vi "剖面多参数上传.vi"(11 "错误输入（无错误）":errorcluster) -> (15 "error out":errorcluster)   [LabVIEW 2016, in "数据传输系统-05.lvlib"]
uses:
  <vilib>/Utility/config.llb/Write Key (String).vi
  <vilib>/Utility/config.llb/Read Key (String).vi
  <vilib>/Utility/config.llb/NI_LVConfig.lvlib
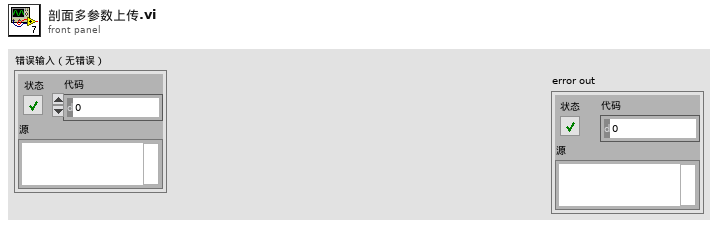
[diagram p1: front panel]
types:
  T1 = cluster{"setini":string, "sysini":string, "hechaini":string, "actualwrite":string, "actualread":string, "datasent":string, "反控命令信息队列":string, "反控与仪器交互":string}
  T2 = typedef "NI_LVConfig.lvlib/Config Data RefNum.ctl" = refnum<k1>
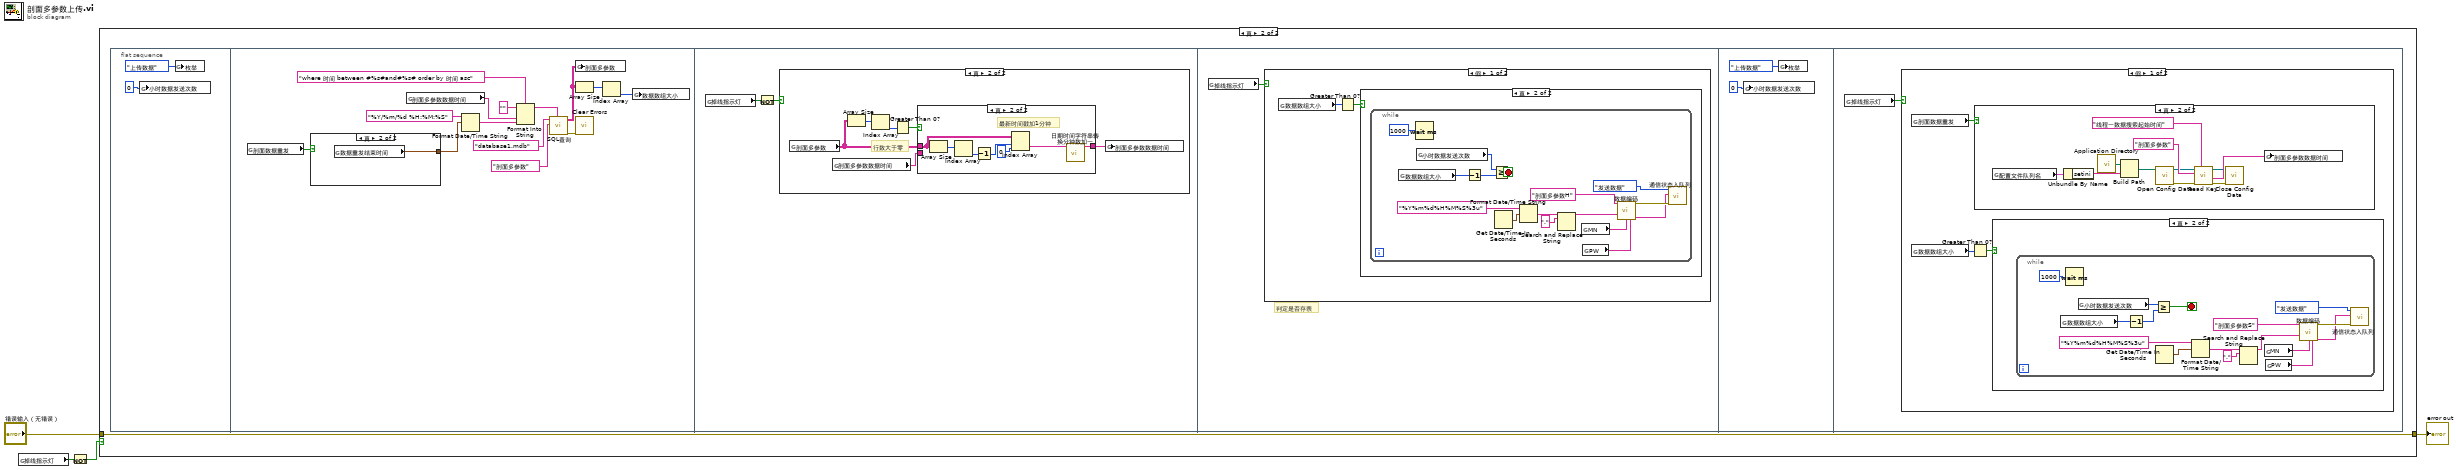
[diagram p0: block diagram]
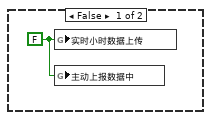
[diagram p2: hidden frame]
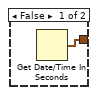
[diagram p3: hidden frame]
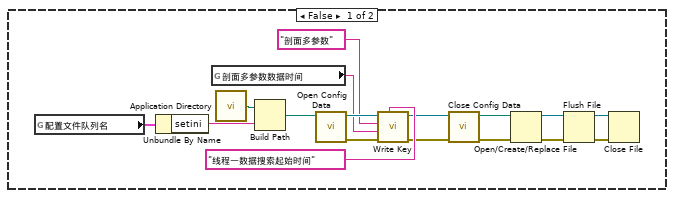
[diagram p8: hidden frame]
diagram:
  n1 = global read "全局 数据发送重叠.vi" "掉线指示灯"() -> (w4:bool)
  n2 = Not(x=w4) -> (.not. x?=w1:bool)
  n3 = case shown="真" w1 {
    tunnel: [_ w6] -> w3
    tunnel: "错误输入（无错误）" -> [_ w6]
    frame False {
      w5 = FALSE ("小时数据上传")
      n4 = global write "全局1.vi" "实时小时数据上传"(w5) -> ()
      n5 = global write "全局 数据发送重叠.vi" "主动上报数据中"(w5) -> ()
    }
    frame True {
      n6 = flat-sequence {
        frame #0 {
          n7 = global write "全局 小时数据发送次数.vi" "小时数据发送次数"(0 ("小时数据发送次数")) -> ()
          n8 = global write "全局1.vi" "枚举"(enum16{"返回请求应答", "上传数据", "返回执行结果"}."上传数据" ("枚举")) -> ()
        }
        frame #1 {
          n9 = global read "断电保存全局.vi" "剖面数据重发"() -> (w10:bool)
          n10 = case shown="真" w10 {
            tunnel: [w23 w24] -> w9
            frame False {
              n11 = Get Date/Time In Seconds() -> (seconds since 1Jan1904=w23:timestamp)
            }
            frame True {
              n12 = global read "断电保存全局.vi" "数据重发结束时间"() -> (w24:timestamp)
            }
          }
          n13 = global read "全局 水样时间.vi" "剖面多参数数据时间"() -> (w17:string)
          n14 = Format Date/Time String(time format string (%c)="%Y/%m/%d %H:%M:%S" ("时间格式字符串(%c)"), seconds (now)=w9) -> (date/time string=w16:string)  [unwired: 1 in]
          n15 = Format Into String(format string="where 时间 between #%s#and#%s# order by 时间 asc" ("condition"), initial string="" ("初始字符串"), w17, w16) -> (resulting string=w15:string)  [unwired: 1 in, 1 out]
          n16 = call "SQL查询.vi"("condition"=w15, "table输入"="剖面多参数", "database"="database1.mdb") -> ("error out"=w11:errorcluster, "data"=w14:string[][])  [unwired: 5 in, 2 out]
          n17 = global write "全局 所有参数.vi" "剖面多参数"(w14) -> ()
          n18 = Array Size(array=w14) -> (size(s)=w13:i32[])
          n19 = call <vilib>:"Clear Errors.vi"("error in (no error)"=w11) -> ()  [unwired: 5 in, 2 out]
          n20 = Index Array(array=w13) -> (element=w12:i32)  [unwired: 1 in]
          n21 = global write "全局 数据数组大小.vi" "数据数组大小"(w12) -> ()
        }
        frame #2 {
          n22 = global read "全局 数据发送重叠.vi" "掉线指示灯"() -> (w26:bool)
          n23 = Not(x=w26) -> (.not. x?=w25:bool)
          n24 = case shown="真" w25 {
            frame False {
            }
            frame True {
              # "行数大于零"
              n25 = global read "全局 所有参数.vi" "剖面多参数"() -> (w31:string[][])
              n26 = global read "全局 水样时间.vi" "剖面多参数数据时间"() -> (w32:string)
              n27 = Array Size(array=w31) -> (size(s)=w28:i32[])
              n28 = Index Array(array=w28) -> (element=w29:i32)  [unwired: 1 in]
              n29 = Greater Than 0?(x=w29) -> (x > 0?=w30:bool)
              n30 = case shown="真" w30 {
                tunnel: w31 -> [_ w37]
                tunnel: [w33 w34] -> w27
                tunnel: w32 -> [w33 _]
                frame False {
                }
                frame True {
                  # "最新时间戳加1分钟"
                  n31 = Array Size(array=w37) -> (size(s)=w39:i32[])
                  n32 = Index Array(array=w39) -> (element=w38:i32)  [unwired: 1 in]
                  n33 = Decrement(x=w38) -> (x-1=w36:i32)
                  n34 = Index Array(array=w37, index (row)=w36, index (col)=0 ("禁用的索引 (列)")) -> (element=w40:string)
                  n35 = call "日期时间字符串转换分钟数加一.vi"("data[0]"=w40) -> ("日期/时间字符串"=w34:string)  [unwired: 10 in]
                }
              }
              n36 = global write "全局 水样时间.vi" "剖面多参数数据时间"(w27) -> ()
            }
          }
        }
        frame #3 {
          # "判定是否存表"
          n37 = global read "全局 数据发送重叠.vi" "掉线指示灯"() -> (w41:bool)
          n38 = case shown="假" w41 {
            frame False {
              n39 = global read "全局 数据数组大小.vi" "数据数组大小"() -> (w42:i32)
              n40 = Greater Than 0?(x=w42) -> (x > 0?=w43:bool)
              n41 = case shown="真" w43 {
                frame False {
                }
                frame True {
                  n42 = while {
                    stop <- w46 stop-if-true
                    n43 = global read "全局 数据数组大小.vi" "数据数组大小"() -> (w48:i32)
                    n44 = Wait (ms)(milliseconds to wait=u32 1000 ("等待时间（毫秒）")) -> ()  [unwired: 1 out]
                    n45 = global read "全局 小时数据发送次数.vi" "小时数据发送次数"() -> (w49:i32)
                    n46 = Decrement(x=w48) -> (x-1=w47:i32)
                    n47 = Greater Or Equal?(x=w49, y=w47) -> (x >= y?=w46:bool)
                    n48 = Get Date/Time In Seconds() -> (seconds since 1Jan1904=w57:timestamp)
                    n49 = Format Date/Time String(time format string (%c)="%Y%m%d%H%M%S%3u" ("时间格式字符串(%c)"), seconds (now)=w57) -> (date/time string=w56:string)  [unwired: 1 in]
                    n50 = Search and Replace String(input string=w56, search string="." ("搜索字符串")) -> (result string=w54:string)  [unwired: 6 in, 3 out]
                    n51 = global read "断电保存全局.vi" "MN"() -> (w53:string)
                    n52 = global read "断电保存全局.vi" "PW"() -> (w52:string)
                    n53 = call "数据编码.vi"("table输入"="剖面多参数H" ("新元素/子数组"), "QN"=w54, "MN"=w53, "PW"=w52) -> ("错误常量"=w51:errorcluster, "通讯包字符串"=w44:string)  [unwired: 10 in]
                    n54 = call "通信状态入队列.vi"("错误输入（无错误）"=w51, "发送报文"=w44, "枚举"=enum16{"打开连接", "发送数据", "读取数据", "数据处理", "关闭连接"}."发送数据") -> ()  [unwired: 8 in, 1 out]
                  }
                }
              }
            }
            frame True {
            }
          }
        }
        frame #4 {
          n55 = global write "全局 小时数据发送次数.vi" "小时数据发送次数"(0 ("小时数据发送次数")) -> ()
          n56 = global write "全局1.vi" "枚举"(enum16{"返回请求应答", "上传数据", "返回执行结果"}."上传数据" ("枚举")) -> ()
        }
        frame #5 {
          n57 = global read "全局 数据发送重叠.vi" "掉线指示灯"() -> (w62:bool)
          n58 = case shown="假" w62 {
            frame False {
              n59 = global read "断电保存全局.vi" "剖面数据重发"() -> (w63:bool)
              n60 = global read "全局 数据数组大小.vi" "数据数组大小"() -> (w65:i32)
              n61 = Greater Than 0?(x=w65) -> (x > 0?=w64:bool)
              n62 = case shown="真" w63 {
                frame False {
                  n63 = global read "断电保存全局.vi" "配置文件队列名"() -> (w67:T1)
                  n64 = Unbundle By Name(w67) -> ("setini"=w66:string)
                  n65 = global read "全局 水样时间.vi" "剖面多参数数据时间"() -> (w68:string)
                  n66 = call <vilib>:"Application Directory.vi"() -> ("Application Directory"=w76:path)
                  n67 = Build Path(base path=w76, name or relative path=w66) -> (appended path=w77:path)
                  n68 = call <vilib>:"Open Config Data.vi"("configuration file path"=w77) -> ("error out"=w79:errorcluster, "refnum"=w78:T2)  [unwired: 8 in, 1 out]
                  n69 = call-poly <vilib>:"Write Key.vi"("section"="线程一数据搜索起始时间", "error in (no error)"=w79, "value"=w68, "key"="剖面多参数", "refnum"=w78) -> ("error out"=w81:errorcluster, "refnum out"=w80:T2)  [unwired: 4 in, 1 out]
                  n70 = call <vilib>:"Close Config Data.vi"("error in (no error)"=w81, "refnum"=w80) -> ("error out"=w69:errorcluster, "file path"=w70:path)  [unwired: 8 in]
                  n71 = Open/Create/Replace File(file path (use dialog)=w70, error in=w69) -> (refnum out=w72:refnum<file>, error out=w71:errorcluster)  [unwired: 4 in, 1 out]
                  n72 = Flush File(refnum=w72, error in=w71) -> (refnum out=w73:refnum<file>, error out=w74:errorcluster)
                  n73 = Close File(refnum=w73, error in=w74) -> ()  [unwired: 2 out]
                }
                frame True {
                  n74 = global read "断电保存全局.vi" "配置文件队列名"() -> (w89:T1)
                  n75 = Unbundle By Name(w89) -> ("setini"=w90:string)
                  n76 = call <vilib>:"Application Directory.vi"() -> ("Application Directory"=w88:path)
                  n77 = Build Path(base path=w88, name or relative path=w90) -> (appended path=w91:path)
                  n78 = call <vilib>:"Open Config Data.vi"("configuration file path"=w91) -> ("error out"=w85:errorcluster, "refnum"=w84:T2)  [unwired: 8 in, 1 out]
                  n79 = call-poly <vilib>:"Read Key.vi"("section"="线程一数据搜索起始时间", "error in (no error)"=w85, "key"="剖面多参数", "refnum"=w84) -> ("error out"=w87:errorcluster, "value"=w93:string, "refnum out"=w86:T2)  [unwired: 4 in, 1 out]
                  n80 = call <vilib>:"Close Config Data.vi"("error in (no error)"=w87, "refnum"=w86) -> ()  [unwired: 8 in, 2 out]
                  n81 = global write "全局 水样时间.vi" "剖面多参数数据时间"(w93) -> ()
                }
              }
              n82 = case shown="真" w64 {
                frame False {
                }
                frame True {
                  n83 = while {
                    stop <- w96 stop-if-true
                    n84 = global read "全局 数据数组大小.vi" "数据数组大小"() -> (w98:i32)
                    n85 = Wait (ms)(milliseconds to wait=u32 1000 ("等待时间（毫秒）")) -> ()  [unwired: 1 out]
                    n86 = global read "全局 小时数据发送次数.vi" "小时数据发送次数"() -> (w99:i32)
                    n87 = Decrement(x=w98) -> (x-1=w97:i32)
                    n88 = Greater Or Equal?(x=w99, y=w97) -> (x >= y?=w96:bool)
                    n89 = Get Date/Time In Seconds() -> (seconds since 1Jan1904=w107:timestamp)
                    n90 = Format Date/Time String(time format string (%c)="%Y%m%d%H%M%S%3u" ("时间格式字符串(%c)"), seconds (now)=w107) -> (date/time string=w106:string)  [unwired: 1 in]
                    n91 = Search and Replace String(input string=w106, search string="." ("搜索字符串")) -> (result string=w104:string)  [unwired: 6 in, 3 out]
                    n92 = global read "断电保存全局.vi" "MN"() -> (w103:string)
                    n93 = global read "断电保存全局.vi" "PW"() -> (w102:string)
                    n94 = call "数据编码.vi"("table输入"="剖面多参数S" ("新元素/子数组"), "QN"=w104, "MN"=w103, "PW"=w102) -> ("错误常量"=w101:errorcluster, "通讯包字符串"=w94:string)  [unwired: 10 in]
                    n95 = call "通信状态入队列.vi"("错误输入（无错误）"=w101, "发送报文"=w94, "枚举"=enum16{"打开连接", "发送数据", "读取数据", "数据处理", "关闭连接"}."发送数据") -> ()  [unwired: 8 in, 1 out]
                  }
                }
              }
            }
            frame True {
            }
          }
        }
      }
    }
  }
  "error out" <- w3
